vi "Launch VIPM Package.vi"(8 "error in (no error)":errorcluster, 11 "VIP File":path) -> (0 "error out":errorcluster)   [LabVIEW 2014]
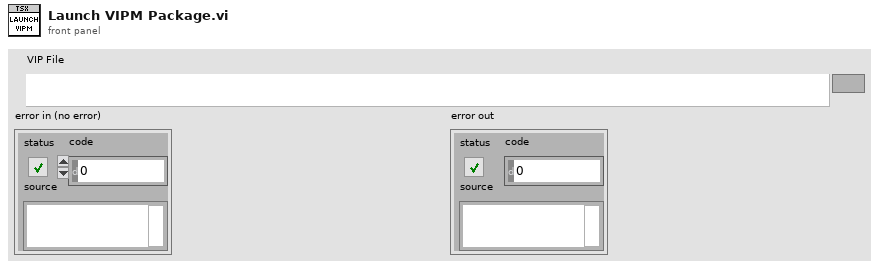
[diagram p1: front panel]
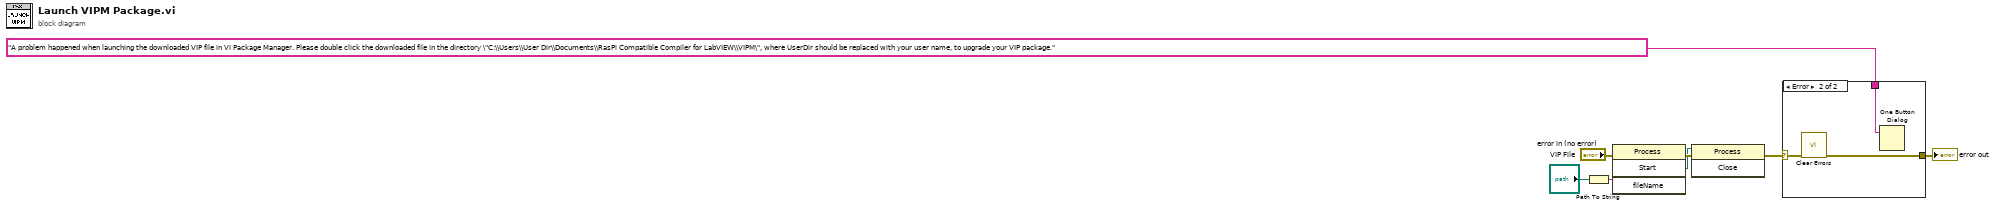
[diagram p0: block diagram]
diagram:
  n1 = Path To String(path="VIP File") -> (string=w7:string)
  n2 = invoke class="Process" method="Start"(error in="error in (no error)", "fileName"=w7) -> (error out=w6:errorcluster, "Start"=w5:refnum<k24>)  [unwired: 2 in, 2 out]
  n3 = invoke class="Process" method="Close"(reference=w5, error in=w6) -> (error out=w3:errorcluster)  [unwired: 1 in, 2 out]
  n4 = case shown="Error" w3 {
    selector: w3 -> [w9 w12]
    tunnel: [w9 w11] -> w1
    tunnel: "A problem happened when launching the downloaded VIP file in VI Package Manager. Please double click the downloaded file in the directory \"C:\\Users\\User Dir\\Documents\\RasPi Compatible Compiler for LabVIEW\\VIPM\", where UserDir should be replaced with your user name, to upgrade your VIP package." ("message") -> [_ w10]
    frame No Error {
    }
    frame Error {
      n5 = call <vilib>:"Clear Errors.vi"("error in (no error)"=w12) -> ("error out"=w11:errorcluster)  [unwired: 5 in, 1 out]
      n6 = One Button Dialog(message=w10) -> ()  [unwired: 1 in, 1 out]
    }
  }
  "error out" <- w1
